vi "Get and write data.vi"() -> ()   [LabVIEW 2013]
uses:
  DAQ_global.vi
panel:
  out "Дата/время":string
  in  "Путь к файлу протокола":path
  in  "Оператор":string="Шляк+Маилян"
  out "Массив данных":dbl[][](array[numeric])
  out "Диаграмма амплитуды":dbl(graph)
  in  "Delay, ms":u32=500
  in  "Число измерений":i32=10
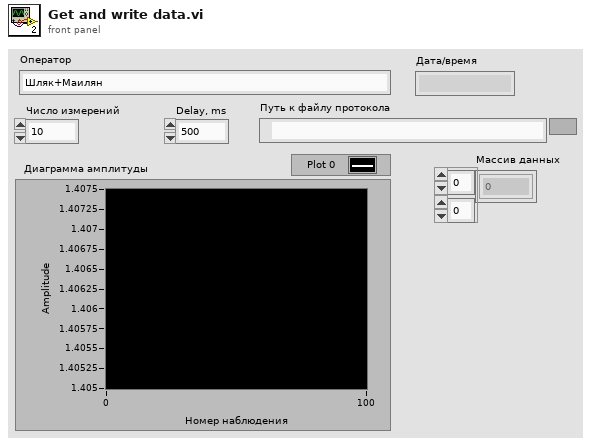
[diagram p1: front panel]
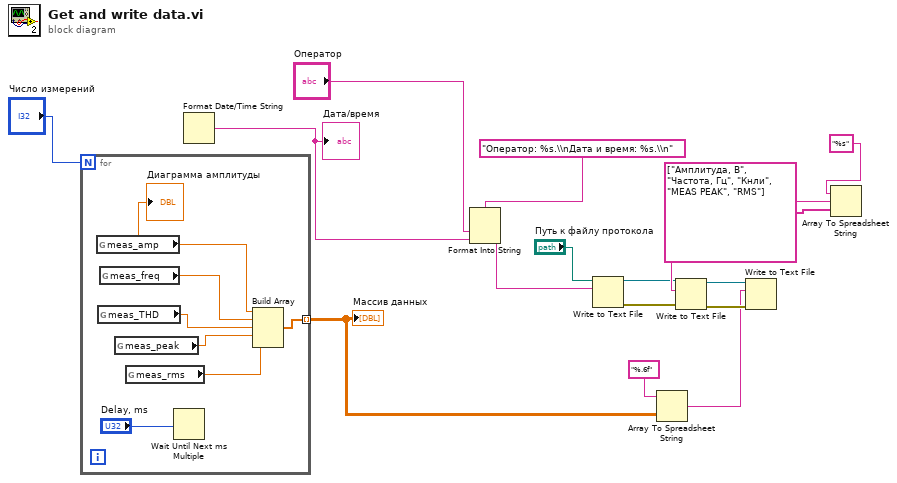
[diagram p0: block diagram]
diagram:
  n1 = for {
    N: "Число измерений" -> [_]
    tunnel: [w19] -> w6 mode=indexing
    n2 = global read "DAQ_global.vi" "meas_amp"() -> (w21:dbl)
    "Диаграмма амплитуды" <- w21
    n3 = global read "DAQ_global.vi" "meas_THD"() -> (w22:dbl)
    n4 = global read "DAQ_global.vi" "meas_freq"() -> (w23:dbl)
    n5 = global read "DAQ_global.vi" "meas_peak"() -> (w18:dbl)
    n6 = global read "DAQ_global.vi" "meas_rms"() -> (w17:dbl)
    n7 = Wait Until Next ms Multiple(millisecond multiple="Delay, ms") -> ()  [unwired: 1 out]
    n8 = Build Array(w21, w23, w22, w18, w17) -> (w19:dbl[])
  }
  "Массив данных" <- w6
  n9 = Format Date/Time String() -> (date/time string=w14:string)  [unwired: 3 in]
  "Дата/время" <- w14
  n10 = Format Into String(format string="Оператор: %s.\\nДата и время: %s.\\n", "Оператор", w14) -> (resulting string=w12:string)  [unwired: 2 in, 1 out]
  n11 = Write to Text File(file (use dialog)="Путь к файлу протокола", text=w12) -> (refnum out=w2:refnum<file>, error out=w9:errorcluster)  [unwired: 2 in, 1 out]
  n12 = Array To Spreadsheet String(array=w6, 3:"%.6f") -> (spreadsheet string=w4:string)  [unwired: 1 in]
  n13 = Array To Spreadsheet String(array=string[] ["Амплитуда, В", "Частота, Гц", "Кнли", "MEAS PEAK", "RMS"], 3:"%s") -> (spreadsheet string=w5:string)  [unwired: 1 in]
  n14 = Write to Text File(file (use dialog)=w2, text=w5, error in=w9) -> (refnum out=w1:refnum<file>, error out=w8:errorcluster)  [unwired: 1 in, 1 out]
  n15 = Write to Text File(file (use dialog)=w1, text=w4, error in=w8) -> ()  [unwired: 1 in, 3 out]
